vi "Analog Output - 1 Channel - Continuous Sampling.vi"() -> ()   [LabVIEW 2019]
uses:
  <vilib>/myRIO/Common/Instrument Driver Framework/myRIO v1.0/UART/vis/myRIO v1.0 Close UART.vi
  <vilib>/myRIO/Instrument Drivers/Onboard IO/AO Continuous/vis/AO Continuous Smart Write.vi
  <vilib>/myRIO/Common/Instrument Driver Framework/Utilities/vis/FPGA Ref Manager.vi
  <vilib>/myRIO/Common/Instrument Driver Framework/ELVIS III v1.0/ELVIS III v1.0 Reset FPGA.vi
  <vilib>/myRIO/Common/Instrument Driver Framework/myRIO v1.0/IRQ/vis/myRIO v1.0 IRQ Info FGV.vi
  <vilib>/myRIO/Common/Instrument Driver Framework/myRIO v1.0/IRQ/vis/myRIO v1.0 Timer IRQ Info FGV.vi
  <vilib>/myRIO/Common/Instrument Driver Framework/myRIO v1.0/IRQ/vis/myRIO v1.0 ISR Agent.vi
  <vilib>/myRIO/Instrument Drivers/Utilities/vis/Reset Index.vi
  <vilib>/myRIO/Common/Instrument Driver Framework/myRIO v1.0/Resource Manager/vis/myRIO v1.0 Block Write Resource Manager.vi
  <vilib>/myRIO/Express VI/Onboard IO/AO/AO Express VI.xnode
  <vilib>/myRIO/Instrument Drivers/Utilities/Utilities.lvlib
  <vilib>/myRIO/Instrument Drivers/Onboard IO/AO Continuous/AO Continuous.lvlib
panel:
  in  "Stop":bool
  in  "A/AO0 (V)":dbl min=-10.0 max=10.0 step=0.1
  # "ELVIS III Control IO"
  # "模拟输出单通道"
  # "Overview: Generates a voltage value on Bank A, Channel AO0 (A/AO0).\nInstructions:\n1. Select a voltage value below.\n2. Connect A/AO0 to the positive lead of the load, and connect AGND to the negative lead of the load. AGND is the ground reference terminal for analog output channels.\n3. Run the VI.\nNote: You can change the AO value while the VI is running."
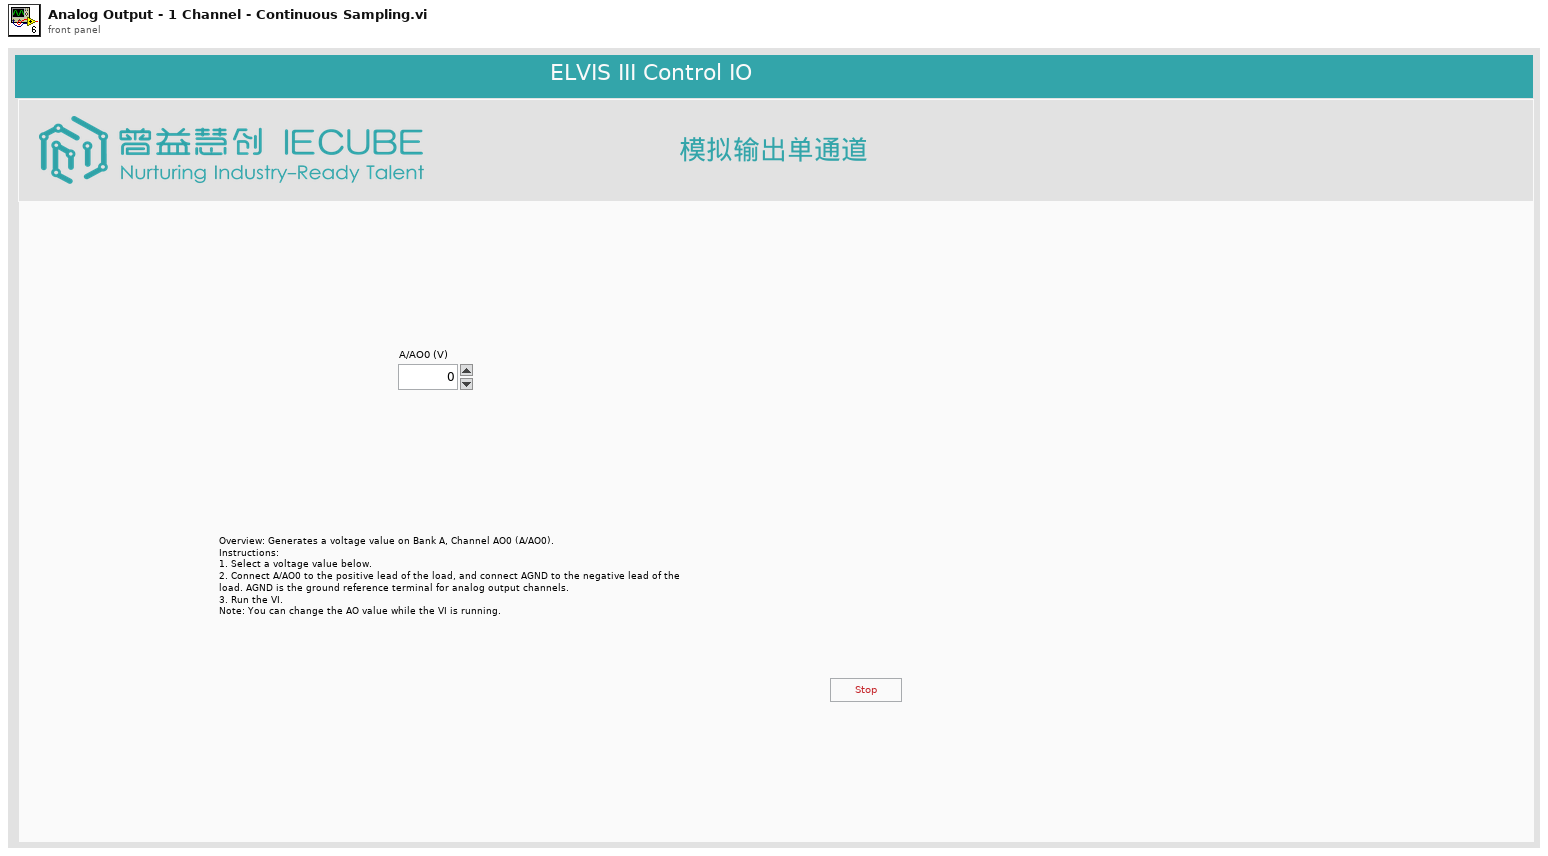
[diagram p1: front panel]
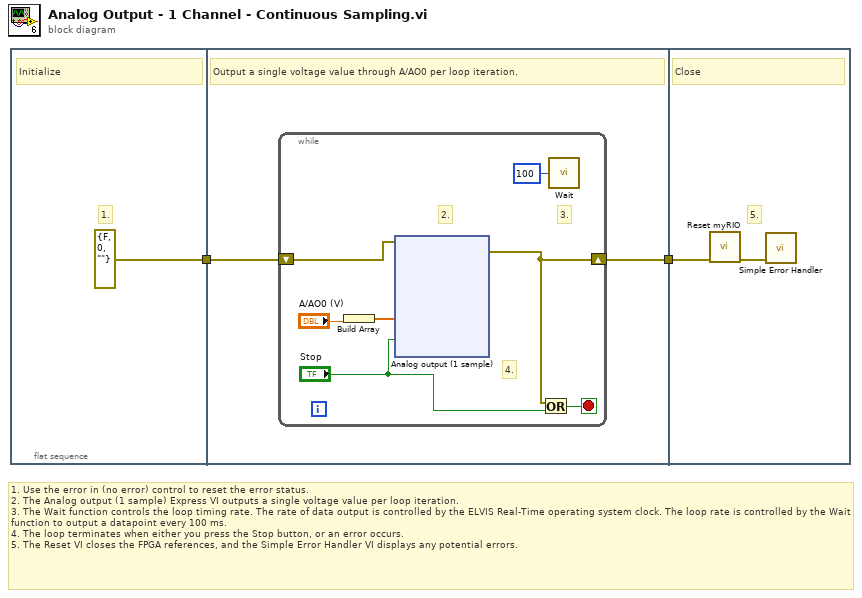
[diagram p0: block diagram]
diagram:
  # "1. Use the error in (no error) control to reset the error status. \n2. The Analog output (1 sample) Express VI outputs a single voltage value per loop iteration.\n3. The Wait function controls the loop timing rate. The rate of data output is controlled by the ELVIS Real-Time operating system clock. The loop rate is controlled by the Wait function to output a datapoint every 100 ms.\n4. The loop terminates when either you press the Stop button, or an error occurs.\n5. The Reset VI closes the FPGA references, and the Simple Error Handler VI displays any potential errors."
  n1 = flat-sequence {
    tunnel: [errorcluster {"status"=FALSE, "code"=0, "source"=""} ("Error In")] -> w2
    tunnel: [w5] -> w1
    tunnel: w2 -> [w4]
    tunnel: w1 -> [w23]
    frame #0 {
      # "1."
      # "Initialize"
    }
    frame #1 {
      # "Output a single voltage value through A/AO0 per loop iteration."
      n2 = while {
        shift-right: [w11] -> w5
        shift-left: w4 -> [w10]
        stop <- w12 stop-if-true
        # "4."
        # "3."
        # "2."
        n3 = Build Array("A/AO0 (V)") -> (w7:dbl[])
        n4 = xnode "Analog output (1 sample)"("A/AO0 (Continuous)"=w7, "Stop?"="Stop", "error in (no error)"=w10) -> ("error out"=w11:errorcluster)
        n5 = Or(x=w11, y="Stop") -> (x .or. y?=w12:bool)
        n6 = call "Wait"("Count(mSec)"=u32 100) -> ()  [unwired: 1 out]
      }
    }
    frame #2 {
      # "5."
      # "Close"
      n7 = call <vilib>:"Reset myRIO.vi"("error in (no error)"=w23) -> ("error out"=w22:errorcluster)  [unwired: 10 in]
      n8 = call <vilib>:"Simple Error Handler.vi"("error in (no error)"=w22) -> ()  [unwired: 4 in, 5 out]
    }
  }
